vi "Plot Line.vi"(6 "Line Plot Config":T1, 7 "module path":path=path "C:/Users/bogum/OneDrive/Dokumenty/Git/LabVIEW Python Ploter/LabVIEW_python_ploter.py", 8 "error in (no error)":errorcluster, 9 "Y":dbl[](array[numeric])=[0.0, 1.0, 2.0, 3.0, 4.0, 5.0, 6.0], 10 "X":dbl[](array[numeric])=[0.0, 1.0, 4.0, 3.0, 3.0, 5.0, 2.0], 11 "PythonPlotter in":refnum<class "PythonPlotter.lvclass">) -> (0 "error out":errorcluster, 3 "PythonPlotter out":refnum<class "PythonPlotter.lvclass">)   [LabVIEW 2024, in "PythonPlotter.lvclass"]
uses:
  PythonPlotter.lvclass
  #linePlotConfig.ctl
  PythonPlotter.lvclass/PythonPlotter.ctl
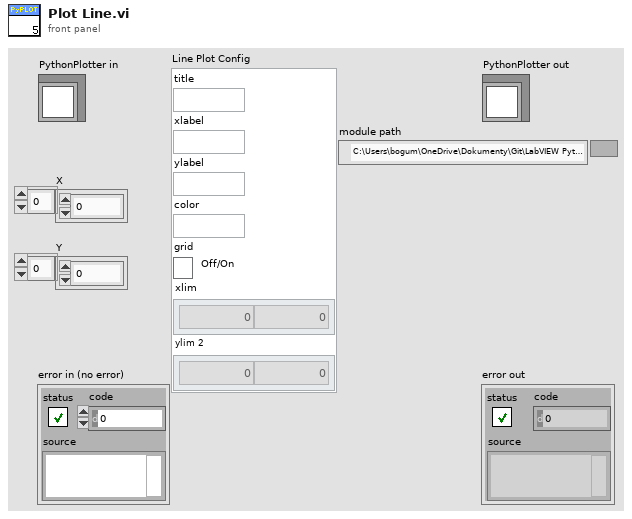
[diagram p1: front panel]
types:
  T1 = typedef "PythonPlotter.lvclass/#linePlotConfig.ctl" = cluster{"title":string, "xlabel":string, "ylabel":string, "color":string, "grid":bool, "xlim":dbl[], "ylim 2":dbl[]}
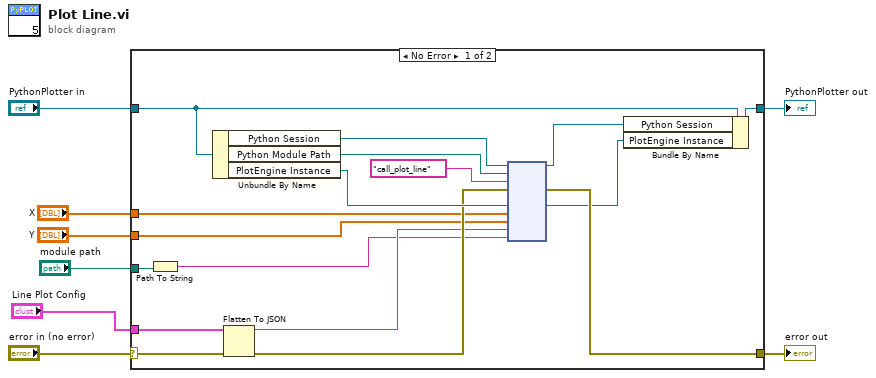
[diagram p0: block diagram]
diagram:
  n1 = case shown="No Error" "error in (no error)" {
    selector: "error in (no error)" -> [w19 w27]
    tunnel: [w12 w27] -> w7
    tunnel: [w11 w26] -> w5
    tunnel: "PythonPlotter in" -> [w25 w26]
    tunnel: "Line Plot Config" -> [w20 _]
    tunnel: "X" -> [w16 _]
    tunnel: "Y" -> [w15 _]
    tunnel: "module path" -> [w14 _]
    frame No Error {
      n2 = Path To String(path=w14) -> (string=w13:string)
      n3 = Unbundle By Name(w25) -> ("Python Session"=w23:refnum<k35>, "Python Module Path"=w22:path, "PlotEngine Instance"=w21:refnum<k38>)
      n4 = Flatten To JSON(anything=w20, error in (no error)=w19) -> (JSON string=w17:string, 11:w18:errorcluster)  [unwired: 1 in]
      n5 = node(w23, w22, "call_plot_line" ("function name"), w18, w21, w16, w15, w17, w13) -> (w10:refnum<k35>, w12:errorcluster, w9:refnum<k38>)  [unwired: 6 in, 2 out]
      n6 = Bundle By Name(cluster=w25, "Python Session"=w10, "PlotEngine Instance"=w9) -> (w11:refnum<class "PythonPlotter.lvclass">)
    }
    frame Error {
    }
  }
  "error out" <- w7
  "PythonPlotter out" <- w5
